vi "IniRead.vi"(7 "section":string caption="段", 8 "error in (no error)":errorcluster caption="错误输入（无错误）", 10 "控件引用":refnum<vi>, 11 "Ini.In":T1 caption="引用句柄") -> (0 "error out":errorcluster caption="错误输出", 3 "Ini.Out":T1 caption="refnum out")   [LabVIEW 2012, in "IniReader&WriterForControl.lvlib"]
uses:
  IniReader&WriterForControl.lvlib
  <vilib>/Utility/config.llb/Config Data RefNum.ctl
  <vilib>/Utility/config.llb/Read Key (String).vi
  <vilib>/Utility/config.llb/Read Key (Double).vi
  <vilib>/Utility/config.llb/Read Key (Path).vi
  <vilib>/Utility/config.llb/Read Key (Boolean).vi
  <vilib>/Utility/config.llb/NI_LVConfig.lvlib
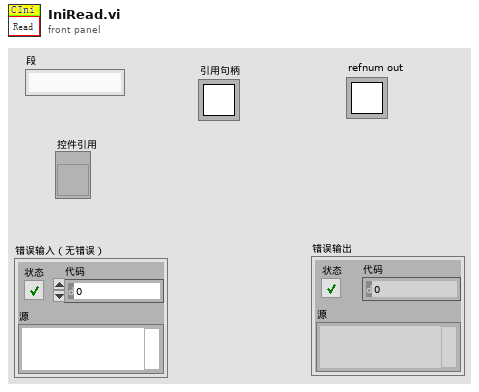
[diagram p1: front panel]
types:
  T1 = typedef "NI_LVConfig.lvlib/Config Data RefNum.ctl" = refnum<k1>
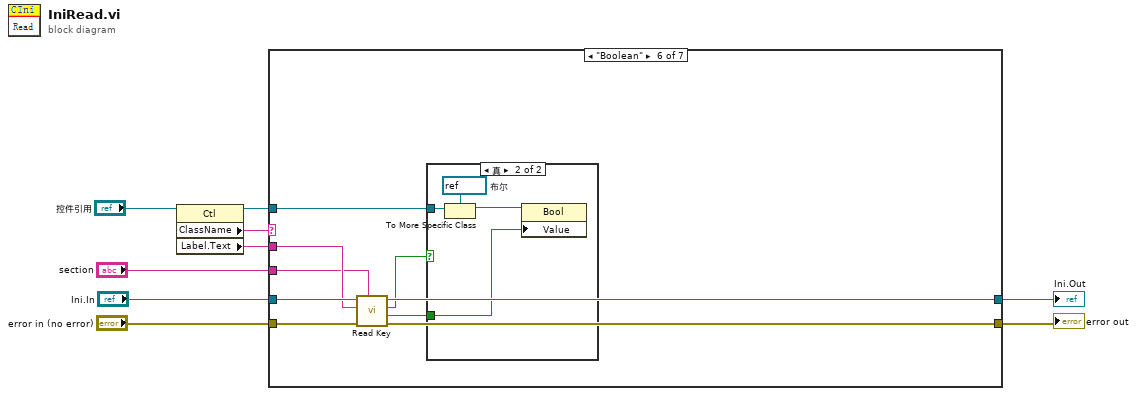
[diagram p0: block diagram]
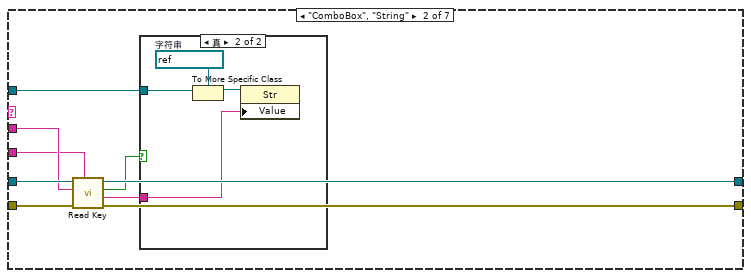
[diagram p3: hidden frame]
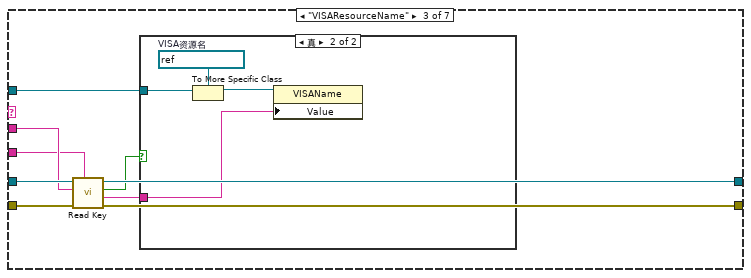
[diagram p5: hidden frame]
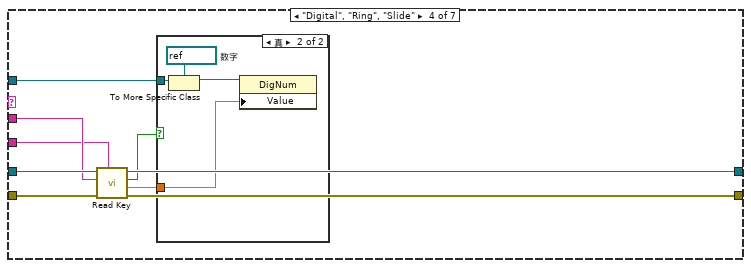
[diagram p7: hidden frame]
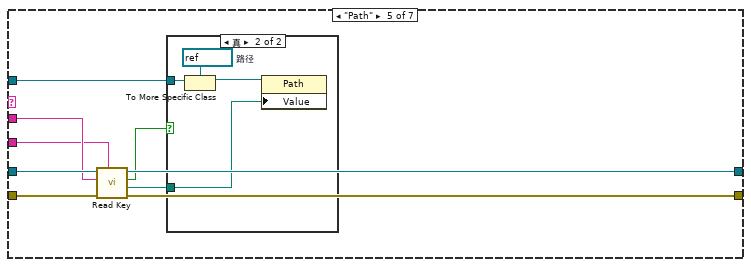
[diagram p9: hidden frame]
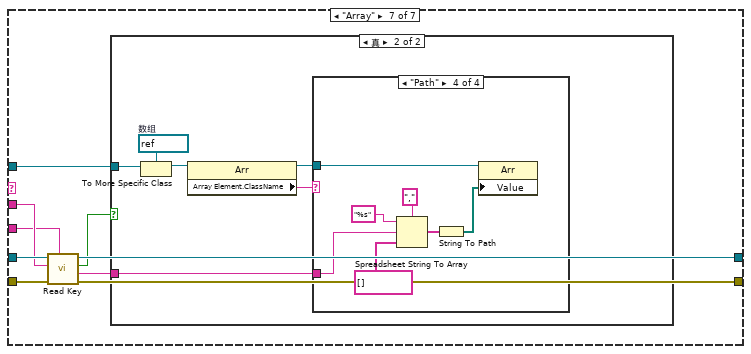
[diagram p12: hidden frame]
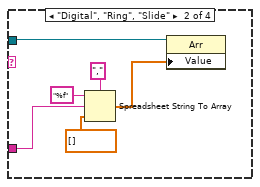
[diagram p15: hidden frame]
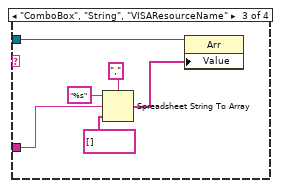
[diagram p16: hidden frame]
diagram:
  n1 = property class="Ctl"(reference="控件引用") -> (reference out=w8:refnum<vi>, "ClassName"=w9:string, "Label.Text"=w6:string)  [unwired: 1 in, 1 out]
  n2 = case shown="\"Boolean\"" w9 {
    tunnel: w8 -> [_ w16 w29 w42 w55 w68 w81]
    tunnel: "Ini.In" -> [w11 w20 w33 w46 w59 w72 w85]
    tunnel: w6 -> [_ w19 w32 w45 w58 w71 w84]
    tunnel: "error in (no error)" -> [w10 w18 w31 w44 w57 w70 w83]
    tunnel: "section" -> [_ w17 w30 w43 w56 w69 w82]
    tunnel: [w10 w14 w27 w40 w53 w66 w80] -> w1
    tunnel: [w11 w13 w26 w39 w52 w65 w79] -> w2
    frame "假", Default {
    }
    frame "ComboBox", "String" {
      n3 = call-poly <vilib>:"Read Key.vi"("section"=w17, "error in (no error)"=w18, "key"=w19, "refnum"=w20) -> ("error out"=w14:errorcluster, "value"=w15:string, "found?"=w12:bool, "refnum out"=w13:T1)  [unwired: 4 in]
      n4 = case shown="真" w12 {
        tunnel: w16 -> [_ w24]
        tunnel: w15 -> [_ w21]
        frame False {
        }
        frame True {
          w23 = refnum<vi> refnum  # 字符串
          n5 = To More Specific Class(target class=w23, reference=w24) -> (specific class reference=w22:refnum<vi>)  [unwired: 1 in, 1 out]
          n6 = property class="Str"(reference=w22, "Value"=w21) -> ()  [unwired: 1 in, 2 out]
        }
      }
    }
    frame "VISAResourceName" {
      n7 = call-poly <vilib>:"Read Key.vi"("section"=w30, "error in (no error)"=w31, "key"=w32, "refnum"=w33) -> ("error out"=w27:errorcluster, "value"=w28:string, "found?"=w25:bool, "refnum out"=w26:T1)  [unwired: 4 in]
      n8 = case shown="真" w25 {
        tunnel: w29 -> [_ w37]
        tunnel: w28 -> [_ w34]
        frame False {
        }
        frame True {
          w36 = refnum<vi> refnum  # VISA资源名
          n9 = To More Specific Class(target class=w36, reference=w37) -> (specific class reference=w35:refnum<vi>)  [unwired: 1 in, 1 out]
          n10 = property class="VISAName"(reference=w35, "Value"=w34) -> ()  [unwired: 1 in, 2 out]
        }
      }
    }
    frame "Digital", "Ring", "Slide" {
      n11 = call-poly <vilib>:"Read Key.vi"("section"=w43, "error in (no error)"=w44, "key"=w45, "refnum"=w46) -> ("error out"=w40:errorcluster, "value"=w41:dbl, "found?"=w38:bool, "refnum out"=w39:T1)  [unwired: 4 in]
      n12 = case shown="真" w38 {
        tunnel: w42 -> [_ w50]
        tunnel: w41 -> [_ w47]
        frame False {
        }
        frame True {
          w49 = refnum<vi> refnum  # 数字
          n13 = To More Specific Class(target class=w49, reference=w50) -> (specific class reference=w48:refnum<vi>)  [unwired: 1 in, 1 out]
          n14 = property class="DigNum"(reference=w48, "Value"=w47) -> ()  [unwired: 1 in, 2 out]
        }
      }
    }
    frame "Path" {
      n15 = call-poly <vilib>:"Read Key.vi"("section"=w56, "error in (no error)"=w57, "key"=w58, "refnum"=w59) -> ("error out"=w53:errorcluster, "value"=w54:path, "found?"=w51:bool, "refnum out"=w52:T1)  [unwired: 4 in]
      n16 = case shown="真" w51 {
        tunnel: w55 -> [_ w63]
        tunnel: w54 -> [_ w60]
        frame False {
        }
        frame True {
          w62 = refnum<vi> refnum  # 路径
          n17 = To More Specific Class(target class=w62, reference=w63) -> (specific class reference=w61:refnum<vi>)  [unwired: 1 in, 1 out]
          n18 = property class="Path"(reference=w61, "Value"=w60) -> ()  [unwired: 1 in, 2 out]
        }
      }
    }
    frame "Boolean" {
      n19 = call-poly <vilib>:"Read Key.vi"("section"=w69, "error in (no error)"=w70, "key"=w71, "refnum"=w72) -> ("error out"=w66:errorcluster, "value"=w67:bool, "found?"=w64:bool, "refnum out"=w65:T1)  [unwired: 4 in]
      n20 = case shown="真" w64 {
        tunnel: w68 -> [_ w76]
        tunnel: w67 -> [_ w73]
        frame False {
        }
        frame True {
          w75 = refnum<vi> refnum  # 布尔
          n21 = To More Specific Class(target class=w75, reference=w76) -> (specific class reference=w74:refnum<vi>)  [unwired: 1 in, 1 out]
          n22 = property class="Bool"(reference=w74, "Value"=w73) -> ()  [unwired: 1 in, 2 out]
        }
      }
    }
    frame "Array" {
      n23 = call-poly <vilib>:"Read Key.vi"("section"=w82, "error in (no error)"=w83, "key"=w84, "refnum"=w85) -> ("error out"=w80:errorcluster, "value"=w77:string, "found?"=w78:bool, "refnum out"=w79:T1)  [unwired: 4 in]
      n24 = case shown="真" w78 {
        tunnel: w81 -> [_ w91]
        tunnel: w77 -> [_ w87]
        frame False {
        }
        frame True {
          w90 = refnum<vi> refnum  # 数组
          n25 = To More Specific Class(target class=w90, reference=w91) -> (specific class reference=w89:refnum<vi>)  [unwired: 1 in, 1 out]
          n26 = property class="Arr"(reference=w89) -> (reference out=w86:refnum<vi>, "Array Element.ClassName"=w88:string)  [unwired: 1 in, 1 out]
          n27 = case shown="\"Path\"" w88 {
            tunnel: w87 -> [_ w94 w99 w106]
            tunnel: w86 -> [_ w93 w98 w107]
            frame "假", Default {
            }
            frame "Digital", "Ring", "Slide" {
              n28 = Spreadsheet String To Array(delimiter (Tab)="," ("分隔符(Tab)"), format string="%f" ("格式字符串"), spreadsheet string=w94, array type (2D Dbl)=dbl[] []) -> (array=w92:dbl[])
              n29 = property class="Arr"(reference=w93, "Value"=w92) -> ()  [unwired: 1 in, 2 out]
            }
            frame "ComboBox", "String", "VISAResourceName" {
              n30 = Spreadsheet String To Array(delimiter (Tab)="," ("分隔符(Tab)"), format string="%s" ("格式字符串"), spreadsheet string=w99, array type (2D Dbl)=string[] []) -> (array=w100:string[])
              n31 = property class="Arr"(reference=w98, "Value"=w100) -> ()  [unwired: 1 in, 2 out]
            }
            frame "Path" {
              n32 = Spreadsheet String To Array(delimiter (Tab)="," ("分隔符(Tab)"), format string="%s" ("格式字符串"), spreadsheet string=w106, array type (2D Dbl)=string[] []) -> (array=w105:string[])
              n33 = String To Path(string=w105) -> (path=w104:path[])
              n34 = property class="Arr"(reference=w107, "Value"=w104) -> ()  [unwired: 1 in, 2 out]
            }
          }
        }
      }
    }
  }
  "error out" <- w1
  "Ini.Out" <- w2
